vi "Create message Queues.vi"(8 "error in":errorcluster) -> (0 "error out":errorcluster, 3 "Messages":T1)   [LabVIEW 2019, in "Messages.lvlib"]
doc: "This VI creates and initializes all the message queues for your application. If your application requires more than one message queue, right-click the \"Message Queues\" constant above and select Open Type Def. Add the new Message Queue(s) to the type definition, then initialize them in this VI."
uses:
  Messages.lvlib
  ctl/Messages.ctl
  <vilib>/NI/AMC/Message Queue.ctl
  <vilib>/NI/AMC/Message.ctl
  <vilib>/NI/Tools/Keyed Array/KeyedArray.ctl
  <vilib>/NI/Tools/Keyed Array/Tools_KeyedArray.lvlib
  <vilib>/NI/AMC/AMC.lvlib
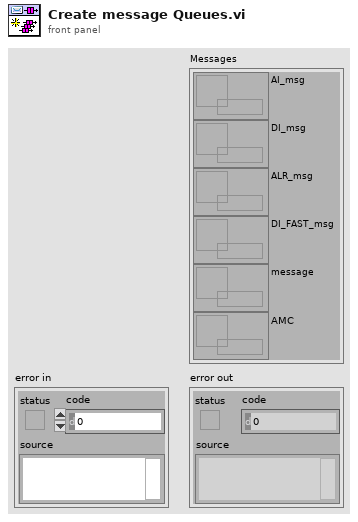
[diagram p1: front panel]
types:
  T1 = typedef "Messages.lvlib/Messages.ctl" = cluster{"AI_msg":refnum<queue>, "DI_msg":refnum<queue>, "ALR_msg":refnum<queue>, "DI_FAST_msg":refnum<queue>, "message":refnum<queue>, "AMC":T2}
  T2 = typedef "AMC.lvlib/Message Queue.ctl" = refnum<queue>
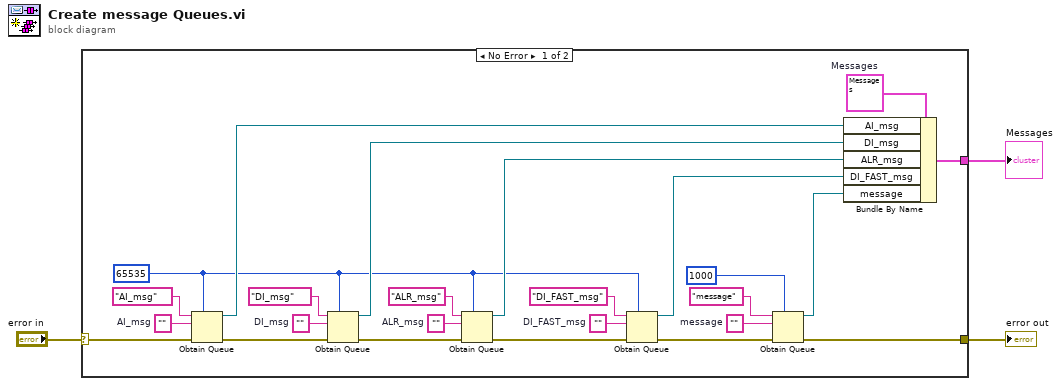
[diagram p0: block diagram]
diagram:
  n1 = case shown="No Error" "error in" {
    selector: "error in" -> [w12 w29]
    tunnel: [w4 w29] -> w3
    tunnel: [w7 _] -> w1
    frame No Error {
      w5 = ""  # message
      w24 = T1 {"AI_msg"=refnum, "DI_msg"=refnum, "ALR_msg"=refnum, "DI_FAST_msg"=refnum, "message"=refnum, "AMC"=refnum}  # Messages
      w22 = ""  # DI_FAST_msg
      w13 = ""  # ALR_msg
      w17 = ""  # DI_msg
      w15 = ""  # AI_msg
      w21 = 65535 ("max queue size (-1, unlimited)")
      n2 = Obtain Queue(max queue size (-1, unlimited)=w21, name (unnamed)="AI_msg", element data type=w15, error in (no error)=w12) -> (queue out=w28:refnum<queue>, error out=w11:errorcluster)  [unwired: 1 in, 1 out]
      n3 = Obtain Queue(max queue size (-1, unlimited)=w21, name (unnamed)="DI_msg", element data type=w17, error in (no error)=w11) -> (queue out=w27:refnum<queue>, error out=w10:errorcluster)  [unwired: 1 in, 1 out]
      n4 = Obtain Queue(max queue size (-1, unlimited)=w21, name (unnamed)="ALR_msg", element data type=w13, error in (no error)=w10) -> (queue out=w26:refnum<queue>, error out=w9:errorcluster)  [unwired: 1 in, 1 out]
      n5 = Obtain Queue(max queue size (-1, unlimited)=w21, name (unnamed)="DI_FAST_msg", element data type=w22, error in (no error)=w9) -> (queue out=w25:refnum<queue>, error out=w8:errorcluster)  [unwired: 1 in, 1 out]
      n6 = Obtain Queue(max queue size (-1, unlimited)=1000, name (unnamed)="message", element data type=w5, error in (no error)=w8) -> (queue out=w6:refnum<queue>, error out=w4:errorcluster)  [unwired: 1 in, 1 out]
      n7 = Bundle By Name(cluster=w24, "AI_msg"=w28, "DI_msg"=w27, "ALR_msg"=w26, "DI_FAST_msg"=w25, "message"=w6) -> (w7:T1)
    }
    frame Error {
    }
  }
  "error out" <- w3
  "Messages" <- w1
